vi "Kill_Errors.vi"(8 "error in (no error)":errorcluster, 11 "refnum in":refnum<file>) -> (0 "error out":errorcluster, 3 "refnum":refnum<file>)   [LabVIEW 2016]
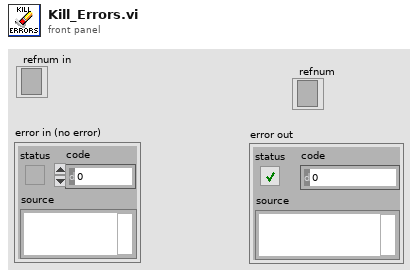
[diagram p1: front panel]
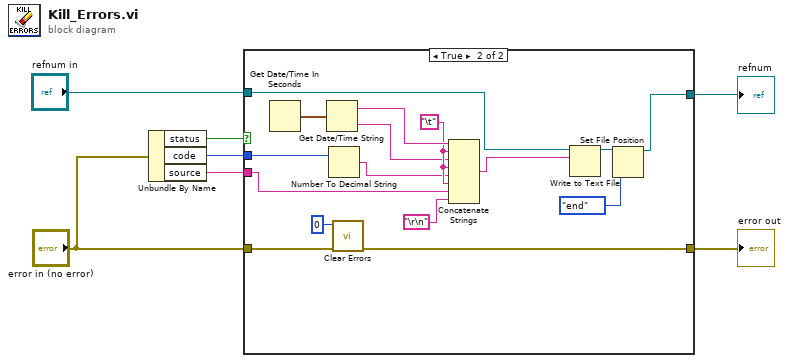
[diagram p0: block diagram]
diagram:
  n1 = Unbundle By Name("error in (no error)") -> ("status"=w7:bool, "code"=w6:i32, "source"=w5:string)
  n2 = case shown="True" w7 {
    tunnel: w6 -> [_ w21]
    tunnel: w5 -> [_ w19]
    tunnel: "error in (no error)" -> [w9 w25]
    tunnel: [w9 w23] -> w3
    tunnel: [w8 w12] -> w2
    tunnel: "refnum in" -> [w8 w10]
    frame False {
    }
    frame True {
      w18 = "\t"
      n3 = Get Date/Time In Seconds() -> (seconds since 1Jan1904=w22:timestamp)
      n4 = Get Date/Time String(seconds (now)=w22) -> (date string=w20:string, time string=w17:string)  [unwired: 2 in]
      n5 = Number To Decimal String(number=w21) -> (decimal integer string=w16:string)  [unwired: 1 in]
      n6 = call <vilib>:"Clear Errors.vi"("error in (no error)"=w25, "specific error code to clear (0: all)"=0) -> ("error out"=w23:errorcluster)  [unwired: 4 in, 1 out]
      n7 = Concatenate Strings(w20, w18, w17, w18, w16, w18, w19, "\r\n") -> (w14:string)
      n8 = Write to Text File(file (use dialog)=w10, text=w14) -> (refnum out=w13:refnum<file>)  [unwired: 2 in, 2 out]
      n9 = Set File Position(refnum=w13, from (0:start)=enum16{"start", "end", "current"}."end") -> (refnum out=w12:refnum<file>)  [unwired: 2 in, 1 out]
    }
  }
  "error out" <- w3
  "refnum" <- w2
